vi "python.vi"() -> ()   [LabVIEW 2018]
panel:
  in  "choose func":enum16{"ready", "camera_start", "inference"}(ring)
  in  "정지 2":bool
  out "에러 출력 2":errorcluster caption="에러 1"
  in  "camera_start":string
  out "result":i32
  in  "정지":bool
  out "에러 출력":errorcluster caption="에러 1"
  in  "inference":string
  in  "python module":path
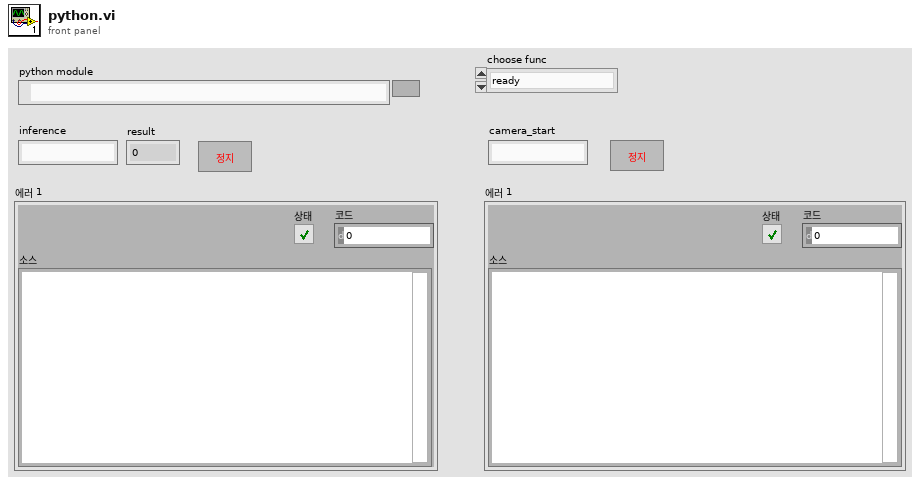
[diagram p1: front panel]
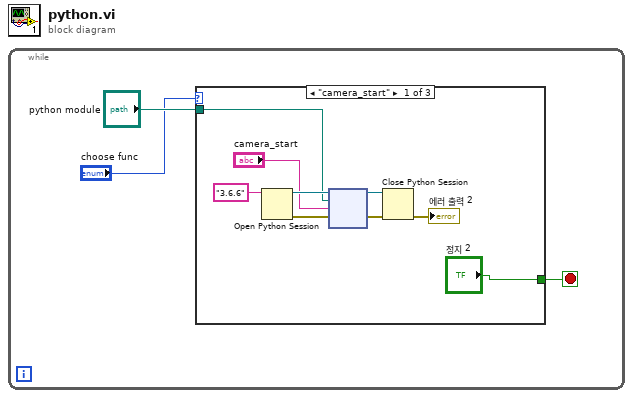
[diagram p0: block diagram]
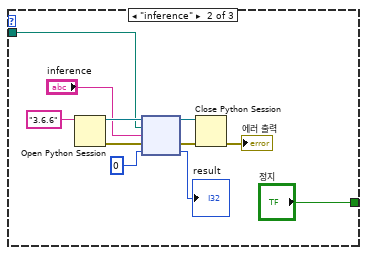
[diagram p2: hidden frame]
diagram:
  n1 = while {
    stop <- w3 stop-if-true
    n2 = case shown="\"camera_start\"" "choose func" {
      tunnel: ["정지 2" "정지" _] -> w3
      tunnel: "python module" -> [w5 w13 _]
      frame "camera_start" {
        n3 = Open Python Session(python version="3.6.6" ("Python 버전")) -> (session out=w10:refnum<k35>, error out=w11:errorcluster)  [unwired: 2 in]
        n4 = node(w10, w5, "camera_start", w11) -> (w7:refnum<k35>, w9:errorcluster)  [unwired: 2 in, 2 out]
        n5 = Close Python Session(session in=w7, error in=w9) -> (11:→"에러 출력 2":errorcluster)
      }
      frame "inference" {
        n6 = Open Python Session(python version="3.6.6" ("Python 버전")) -> (session out=w19:refnum<k35>, error out=w20:errorcluster)  [unwired: 2 in]
        n7 = node(w19, w13, "inference", w20, 0) -> (w16:refnum<k35>, w18:errorcluster, →"result":i32)  [unwired: 2 out]
        n8 = Close Python Session(session in=w16, error in=w18) -> (11:→"에러 출력":errorcluster)
      }
      frame "ready" {
      }
    }
  }
